vi "Time_Trigger.vi"() -> ()   [LabVIEW 2020]
panel:
  in  "Time_trigger":bool
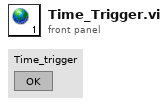
[diagram p1: front panel]
diagram:
